vi "Write INI Cluster.vi"(5 "float number format (optional)":string, 8 "error in (no error)":errorcluster, 10 "INI Fomatted Cluster":variant, 11 "refnum":T1) -> (0 "error out":errorcluster, 3 "dup refnum":T1)   [LabVIEW 2017, in "OpenG Variant Configuration File.lvlib"]
doc: "Writes a cluster of section formatted clusters to configuration data identified by refnum. Section cluster names are used as section names and key-value pairs correspond to the named cluster elements and thier values within the section formatted clusters. Only the items within the \"INI Formatted Cluster\" input cluster are written to the configuration data.\n\nFor example an Cluster containins subClusters MyCluster1 and MyCluster2, where MyCluster1 contains two elements MyNumeric and MyBoolean, and MyCluster2 contains two elements MyEnum and MyString. This would correspond to an INI write of the following data:\n\n[MyCluster1]\nMyNumeric=1.024\nMyBoolean=TRUE\n[MyCluster2]\nMyEnum=init\nMyString=\"Hello World\"\n\nNote: Special characters in section and key names will be escape-coded. These include the following: \\00-\\1F (non-printable chars); \"[\", \"]\", and \"=\" (INI syntax elements); \\FE (\"þ\") and \\FF (\"ÿ\") (legacy bracket encoding); Additionally, the escape character, \"\\\", will be escaped as \"\\\\\".\n\nNote: This VI checks whether every element of the cluster has a name so it can be identified."
uses:
  OpenG Variant Configuration File.lvlib
  <vilib>/Utility/config.llb/Config Data RefNum.ctl
  _openG/_reuse_openG.lvlib
  <vilib>/Utility/Data Type/NI_Data Type.lvlib
  <vilib>/Utility/config.llb/NI_LVConfig.lvlib
panel:
  # "Write INI Cluster.vi\n\nWrites a cluster (variant) of INI section clusters to INI file.\n\nPlease visit http://www.OpenG.org to learn about the\nOpen Source LabVIEW software movement.\n\nNOTICE -- YOU MUST LEAVE THIS NOTICE IN PLACE.  PER THE TERMS OF THE LICENSE BELOW, YOU MAY SUBLICENSE THIS SOFTWARE \nIN ANY WAY THAT DOES NOT CONFLICT WITH THIS LICENSE.\n\n### BSD License (http://www.opensource.org/licenses/bsd-license.php) Begin ###\n \nCopyright (c) 2002-2006, Jim Kring <jim@jimkring.com>\n\nAll rights reserved.\n\nRedistribution and use in source and binary forms, with or without modification, are permitted provided that the following conditions are met:\n\n    * Redistributions of source code must retain the above copyright notice, this list of conditions and the following disclaimer.\n    * Redistributions in binary form must reproduce the above copyright notice, this list of conditions and the following disclaimer in the \n       documentation and/or other materials provided with the distribution.\n    * Neither the name of SciWare, James Kring, Inc., nor the names of its contributors may be used to endorse or promote products derived \n       from this software without specific prior written permission.\n\nTHIS SOFTWARE IS PROVIDED BY THE COPYRIGHT HOLDERS AND CONTRIBUTORS \"AS IS\" AND ANY EXPRESS OR IMPLIED WARRANTIES, \nINCLUDING, BUT NOT LIMITED TO, THE IMPLIED WARRANTIES OF MERCHANTABILITY AND FITNESS FOR A PARTICULAR PURPOSE ARE \nDISCLAIMED. IN NO EVENT SHALL THE COPYRIGHT OWNER OR CONTRIBUTORS BE LIABLE FOR ANY DIRECT, INDIRECT, INCIDENTAL,\n SPECIAL, EXEMPLARY, OR CONSEQUENTIAL DAMAGES (INCLUDING, BUT NOT LIMITED TO, PROCUREMENT OF SUBSTITUTE GOODS OR \nSERVICES; LOSS OF USE, DATA, OR PROFITS; OR BUSINESS INTERRUPTION) HOWEVER CAUSED AND ON ANY THEORY OF LIABILITY, \nWHETHER IN CONTRACT, STRICT LIABILITY, OR TORT (INCLUDING NEGLIGENCE OR OTHERWISE) ARISING IN ANY WAY OUT OF THE USE \nOF THIS SOFTWARE, EVEN IF ADVISED OF THE POSSIBILITY OF SUCH DAMAGE.\n\n### BSD License End ###"
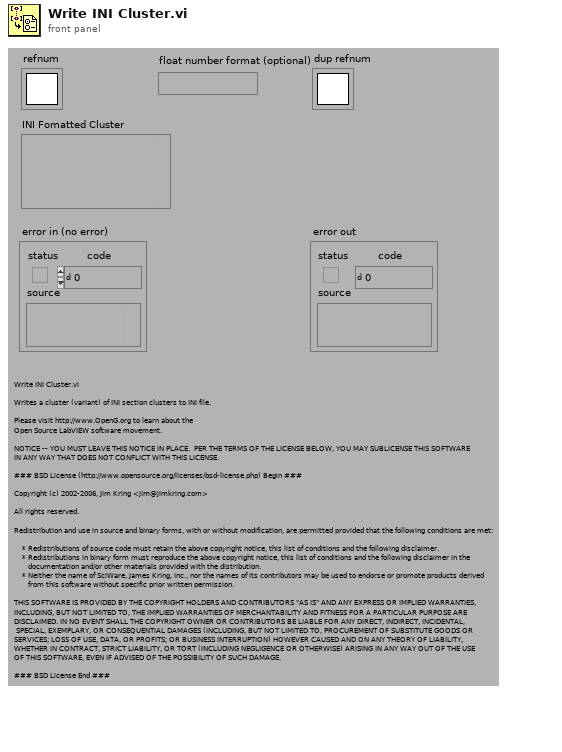
[diagram p1: front panel]
types:
  T1 = typedef "NI_LVConfig.lvlib/Config Data RefNum.ctl" = refnum<k1>
  T2 = typedef "NI_Data Type.lvlib/Data Type.ctl" = enum8{"Invalid Type", "Void", "I8", "I16", "I32", "I64", "U8", "U16", "U32", "U64", "Single Float", "Double Float", "Extended Float", "Single Complex", "Double Complex", "Extended Complex", "Enum U8", "Enum U16", "Enum U32", "Enum U64", "Single Float With Unit", "Double Float With Unit", "Extended Float With Unit", "Single Complex with Unit", "Double Complex with Unit", "Extended Complex with Unit", "Boolean", "String", "Path", "Picture", "Tag", "Array", "Cluster", "Variant", "LV Variant", "Waveform", "Timestamp", "Digital Waveform", "Digital Data", "ExpressData", "Refnum", "External Data", "VI", "Poly VI", "LabVIEW Class Instance", "Fixed Point"}
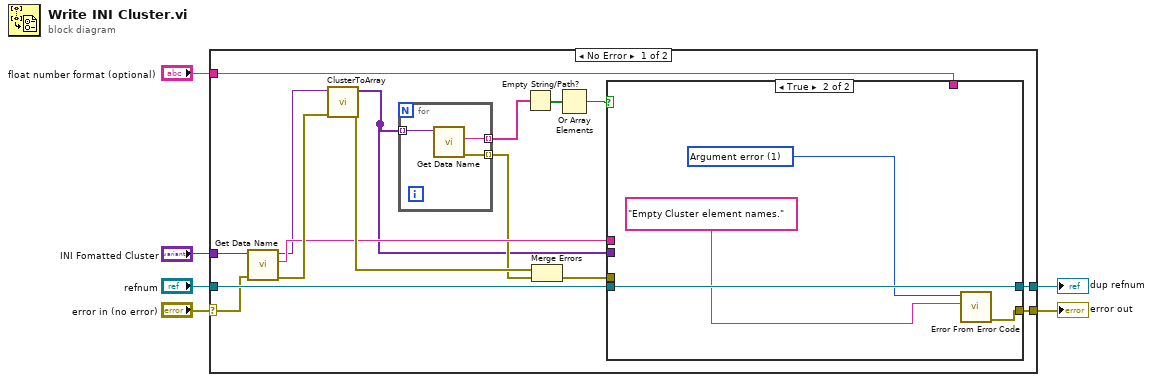
[diagram p0: block diagram]
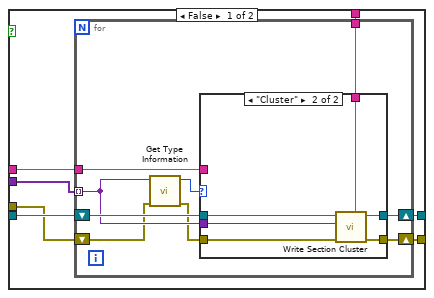
[diagram p2: hidden frame]
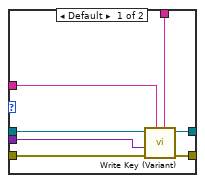
[diagram p3: hidden frame]
diagram:
  n1 = case shown="No Error" "error in (no error)" {
    selector: "error in (no error)" -> [w17 w60]
    tunnel: [w22 w60] -> w6
    tunnel: [w21 w59] -> w5
    tunnel: "refnum" -> [w20 w59]
    tunnel: "INI Fomatted Cluster" -> [w19 _]
    tunnel: "float number format (optional)" -> [w18 _]
    frame No Error {
      n2 = call "Get Data Name.vi"("error in (no error)"=w17, "Data"=w19) -> ("error out"=w16:errorcluster, "Data Name"=w14:string, "Data Dup"=w12:variant)  [unwired: 7 in]
      n3 = call "ClusterToArray.vi"("Error in"=w16, "Cluster"=w12) -> ("Error out"=w15:errorcluster, "Array"=w7:variant[])  [unwired: 8 in]
      n4 = for {
        tunnel: w7 -> [w25] mode=indexing
        tunnel: [w24] -> w9 mode=indexing
        tunnel: [w23] -> w8 mode=indexing
        n5 = call "Get Data Name.vi"("Data"=w25) -> ("error out"=w23:errorcluster, "Data Name"=w24:string)  [unwired: 8 in, 1 out]
      }
      n6 = Empty String/Path?(string/path=w9) -> (empty?=w13:bool[])
      n7 = Merge Errors(w15, w8) -> (w10:errorcluster)
      n8 = Or Array Elements(Boolean array=w13) -> (logical OR=w11:bool)
      n9 = case shown="True" w11 {
        tunnel: [w32 w57] -> w22
        tunnel: [w31 w58] -> w21
        tunnel: w20 -> [w30 w58]
        tunnel: w18 -> [w29 _]
        tunnel: w10 -> [w27 _]
        tunnel: w14 -> [w28 _]
        tunnel: w7 -> [w26 _]
        frame False {
          n10 = for {
            tunnel: w26 -> [w38] mode=indexing
            shift-right: [w39] -> w31
            shift-left: w30 -> [w41]
            shift-right: [w40] -> w32
            shift-left: w27 -> [w34]
            tunnel: w28 -> [w36]
            tunnel: w29 -> [w35]
            n11 = call <vilib>:"Get Type Information.vi"("error in (no error)"=w34, "Variant"=w38) -> ("error out"=w33:errorcluster, "Type"=w37:T2)  [unwired: 5 in, 3 out]
            n12 = case shown="\"Cluster\"" w37 {
              tunnel: w41 -> [w46 w54]
              tunnel: w33 -> [w48 w53]
              tunnel: [w47 w52] -> w40
              tunnel: [w45 w51] -> w39
              tunnel: w38 -> [w43 w50]
              tunnel: w36 -> [w44 _]
              tunnel: w35 -> [w42 w49]
              frame Default {
                n13 = call "Write Key (Variant).vi"("float number format"=w42, "section"=w44, "error in (no error)"=w48, "key-value"=w43, "refnum"=w46) -> ("error out"=w47:errorcluster, "refnum out"=w45:T1)  [unwired: 5 in]
              }
              frame "Cluster" {
                n14 = call "Write Section Cluster.vi"("float number format (optional)"=w49, "error in (no error)"=w53, "Section Formatted Cluster"=w50, "refnum"=w54) -> ("error out"=w52:errorcluster, "dup refnum"=w51:T1)  [unwired: 6 in]
              }
            }
          }
        }
        frame True {
          w56 = 1 items=["No error", "Argument error", "Memory is full", "Out of zone", "End of file", "File already open", "Generic file I/O error", "File not found", "File permission error", "Disk is full", "Duplicate path", "Too many files open", "System feature not enabled", "Resource file not found", "Cannot add resource", "Resource not found", "Image not found", "Image memory error", "Pen does not exist", "Config type invalid", "Config token not found", "Config parse error", "Config memory error", "Bad external code format", "Bad external code offset", "External code not present", "Null window", "Destroy window error", "Null menu", "Print aborted", "Bad print record", "Print driver error", "Windows error during printing", "Memory error during printing", "Print dialog error", "Generic print error", "Invalid device refnum", "Device not found", "Device parameter error", "Device unit error", "Cannot open device", "Device call aborted", "Generic error", "Cancelled by user", "Object ID too low", "Object ID too high", "Object not in heap", "Unknown heap", "Unknown object (invalid DefProc)", "Unknown object (DefProc not in table)", "Message out of range", "Invalid (null) method", "Unknown message", "Manager call not supported", "Bad address", "Network operation in progress", "Network operation timed out", "Connection is busy", "Network attribute not supported", "Network error", "Address in use", "System out of memory", "Connection aborted", "Connection refused", "Not connected", "Already connected", "Connection closed", "Initialization error (interapplication manager)", "Bad occurrence", "Wait on unbound occurrence handler", "Occurrence queue overflow", "Datalog type conflict", "Unused", "Unrecognized type (interapplication manager)", "Memory corrupt", "Failed to make temporary DLL", "Old CIN version", "Drag socket not found", "Failed to load drop-object", "Failed to register OLE object", "Failed to release OLE object", "Format specifier type mismatch", "Unknown format specifier", "Too few format specifiers", "Too many format specifiers", "Scan failed", "Newer CIN version", "Error converting to variant", "Runtime menu error", "Password tampered", "Variant attribute not found", "Incompatible variant data type", "Event data is not available", "Event Store is not present", "Occurrence is not found", "Event Queue is not created", "Event info is not available", "Refnum passed is NULL", "Error retrieving Class GUID", "Error retrieving CoClass GUID", "Error retrieving TypeLib GUID.", "Bad built application magic bytes.", "Specific driver is different from the specific driver associated with the Logical Name.", "There is no session opened to the class driver.", "Max Error", "MAX - Error with config objects", "MAX - Error loading configuration", "MAX - Group not supported"]
          n15 = call "Error From Error Code.vi"("error message (\"\")"="Empty Cluster element names." ("String to Prepend to source (\"\")"), "error code (0)"=w56) -> ("error out"=w57:errorcluster)  [unwired: 7 in]
        }
      }
    }
    frame Error {
    }
  }
  "error out" <- w6
  "dup refnum" <- w5
